vi "Configure Waveform Modulation (FM).vi"(6 "FM Frequency (1000 Hz)":dbl=1000.0, 8 "error in (no error)":errorcluster, 9 "FM Frequency Deviation (1000 Hz)":dbl=1000.0, 10 "Waveform Generator Number (1: Waveform Generator 1)":i32(ring)=1 items=["Waveform Generator 1"=1], 11 "VISA resource name":refnum<visa-resource-name>) -> (0 "error out":errorcluster, 3 "VISA resource name out":refnum<visa-resource-name>)   [LabVIEW 2010, in "Agilent 2000 3000 X-Series.lvlib"]
doc: "Configures the waveform modulation FM."
uses:
  <instrlib>/Agilent 2000 3000 X-Series/Agilent 2000 3000 X-Series.lvlib
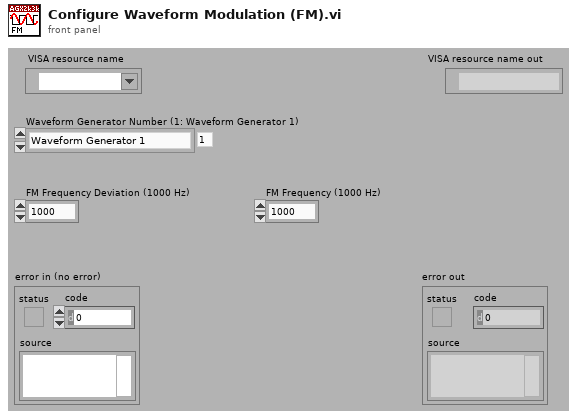
[diagram p1: front panel]
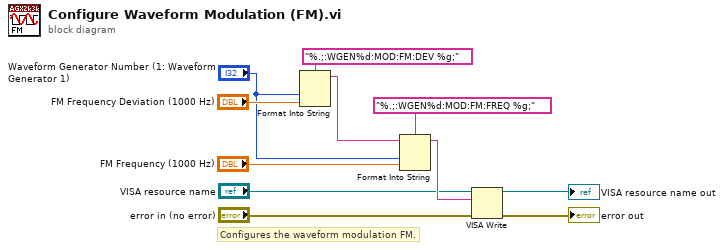
[diagram p0: block diagram]
diagram:
  # "Configures the waveform modulation FM."
  n1 = Format Into String(format string="%.;:WGEN%d:MOD:FM:DEV %g;", "Waveform Generator Number (1: Waveform Generator 1)", "FM Frequency Deviation (1000 Hz)") -> (resulting string=w9:string)  [unwired: 2 in, 1 out]
  n2 = Format Into String(format string="%.;:WGEN%d:MOD:FM:FREQ %g;", initial string=w9, "Waveform Generator Number (1: Waveform Generator 1)", "FM Frequency (1000 Hz)") -> (resulting string=w3:string)  [unwired: 1 in, 1 out]
  n3 = VISA Write(VISA resource name="VISA resource name", write buffer=w3, error in (no error)="error in (no error)") -> (VISA resource name out=→"VISA resource name out":refnum<visa-resource-name>, error out=→"error out":errorcluster)  [unwired: 1 out]
